vi "Untitled 8.vi"() -> ()   [LabVIEW 2016]
uses:
  <vilib>/Analysis/6fits.llb/Curve Fitting Criteria.ctl
  <vilib>/Analysis/NI_AALPro.lvlib
panel:
  out "Data section you choose 2":cluster{dbl[], "Best Polynomial Fit":dbl[]}[](graph)
  in  "Array":dbl[](array[numeric])=[3.0, 4.0, 5.0]
  in  "Data section you choose":cluster{dbl[], "Best Polynomial Fit":dbl[]}[](graph)=[{array[4999 elements], "Best Polynomial Fit"=array[4999 elements]}]
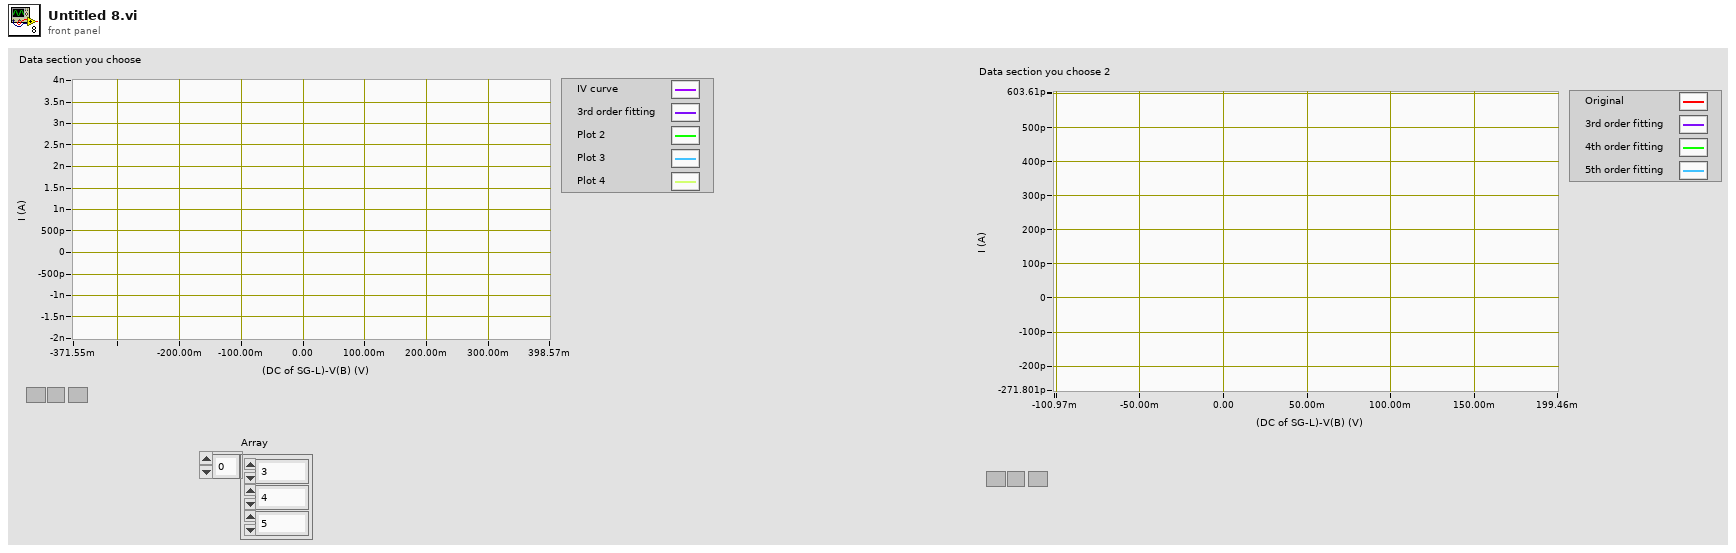
[diagram p1: front panel]
types:
  T1 = typedef "NI_AALPro.lvlib/Curve Fitting Criteria.ctl" = u16
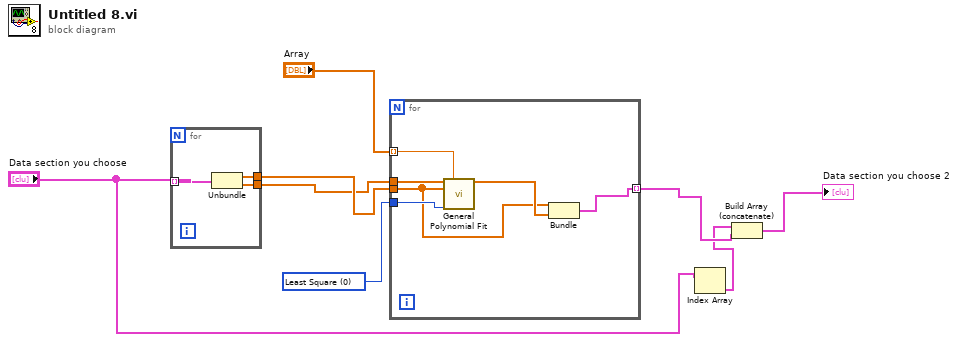
[diagram p0: block diagram]
diagram:
  w5 = T1 0 items=["Least Square", "Least Absolute Residual", "Bisquare"] ("method")
  n1 = for {
    tunnel: "Data section you choose" -> [w11] mode=indexing
    tunnel: [w10] -> w8
    tunnel: [w9] -> w7
    n2 = Unbundle(w11) -> (w10:dbl[], "Best Polynomial Fit"=w9:dbl[])
  }
  n3 = for {
    tunnel: w8 -> [w12]
    tunnel: w7 -> [w16]
    tunnel: "Array" -> [w17] mode=indexing
    tunnel: [w15] -> w2 mode=indexing
    tunnel: w5 -> [w14]
    n4 = call <vilib>:"General Polynomial Fit.vi"("Y"=w16, "polynomial order"=w17, "X"=w12, "method"=w14) -> ("Best Polynomial Fit"=w13:dbl[])  [unwired: 8 in, 3 out]
    n5 = Bundle(w12, "Best Polynomial Fit"=w13) -> (w15:cluster{dbl[], "Best Polynomial Fit":dbl[]})  [unwired: 1 in]
  }
  n6 = Index Array(array="Data section you choose") -> (element=w1:cluster{dbl[], "Best Polynomial Fit":dbl[]})  [unwired: 1 in]
  n7 = Build Array (concatenate)(w1, w2) -> (→"Data section you choose 2":cluster{dbl[], "Best Polynomial Fit":dbl[]}[])
